vi "JoystickSquare.vi"(11 "JoyStickInput":dbl) -> (3 "SquaredOutput":dbl)   [LabVIEW 2023]
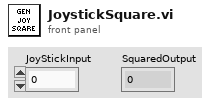
[diagram p1: front panel]
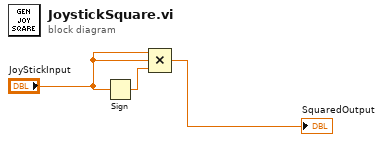
[diagram p0: block diagram]
diagram:
  n1 = Sign(1:"JoyStickInput") -> (0:w2:dbl)
  n2 = Compound Arithmetic op=MULTIPLY("JoyStickInput", "JoyStickInput", w2) -> (→"SquaredOutput":dbl)
